vi "CODCr数据插入DATA (子VI).vi"(11 "Enum输入":refnum<vi>) -> (3 "data":T1)   [LabVIEW 2016, in "CODCr库.lvlib"]
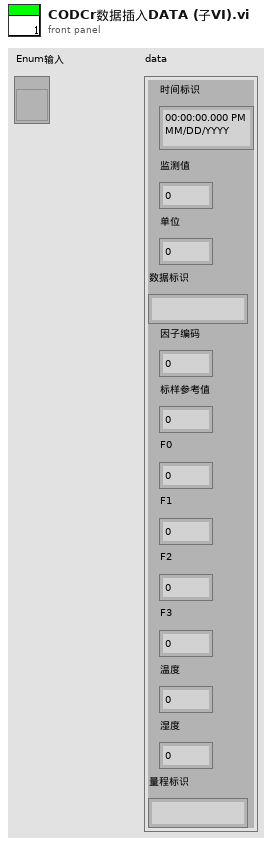
[diagram p1: front panel]
types:
  T1 = cluster{"时间标识":timestamp, "监测值":sgl, "单位":u16, "数据标识":string, "因子编码":u32, "标样参考值":sgl, "F0":sgl, "F1":sgl, "F2":sgl, "F3":sgl, "温度":sgl, "湿度":sgl, "量程标识":string}
  T2 = cluster{"系统时间":timestamp, "工作状态":u16, "测量模式":u16, "告警代码":enum16{"无告警", "缺试剂告警", "缺水样告警", "缺蒸馏水告警", "缺标液告警", "仪表漏液告警", "标定异常告警", "超量程告警", "加热异常", "低试剂预警", "超上限告警", "超下限告警", "仪表内部其他异常", "滴定异常告警", "电极异常告警", "量程切换告警", "参数设置告警", "PH电极电位异常", "电导率电极异常", "浊度光度异常", "溶解氧电极异常", "溶解氧光强异常", "温度异常告警", "PH异常告警", "溶解氧异常告警", "电导率异常告警", "浊度异常告警", "叶绿素异常告警", "藻密度异常告警", "蓝绿藻异常告警", "ORP异常告警", "氨氮异常告警", "清洁刷异常告警", "SD卡异常告警", "蓝牙异常告警", "Wifi异常告警", "流程异常告警"}, "故障代码":enum16{"无故障", "电机故障", "温度故障", "通讯故障", "滴定故障"}, "日志代码":u16, "软件版本":u16, "F0":sgl, "F1":sgl, "F2":sgl, "F3":sgl, "T":sgl, "H":sgl, "id":u16, "flowid":u16, "量程":u16}
  T3 = cluster{"因子编码":u32, "单位":u16, "标样参考值":sgl, "水样数据时间":timestamp, "水样实测值":sgl, "水样数据标识":string, "标样数据时间":timestamp, "标样实测值":sgl, "标样数据标识":string, "空白数据时间":timestamp, "空白实测值":sgl, "空白数据标识":string, "零点核查数据时间":timestamp, "零点核查实测值":sgl, "零点核查数据标识":string, "跨度核查数据时间":timestamp, "跨度核查实测值":sgl, "跨度核查数据标识":string, "加标回收数据时间":timestamp, "加标回收实测值":sgl, "加标回收数据标识":string, "平行样数据时间":timestamp, "平行样实测值":sgl, "平行样数据标识":string}
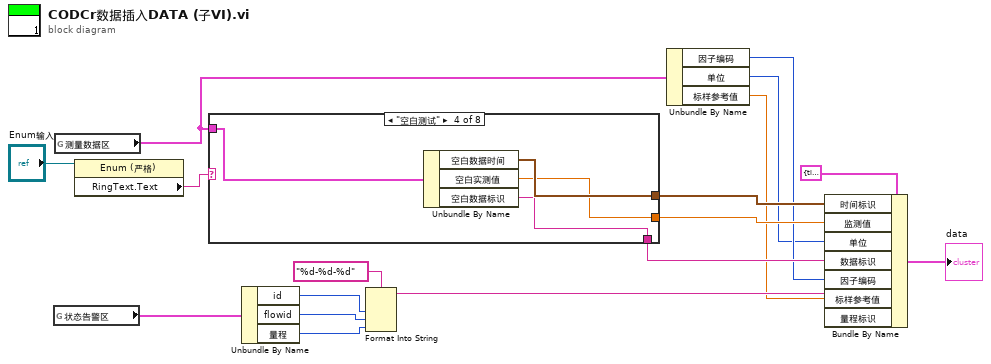
[diagram p0: block diagram]
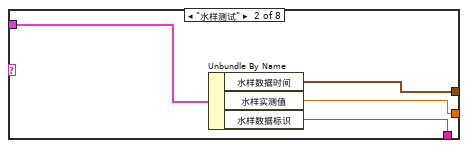
[diagram p3: hidden frame]
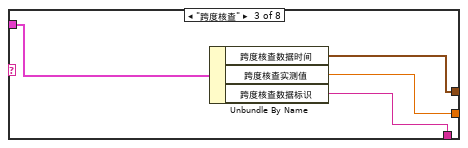
[diagram p4: hidden frame]
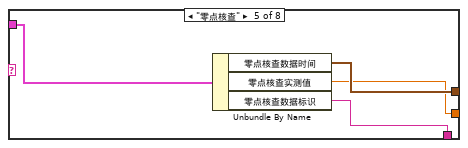
[diagram p5: hidden frame]
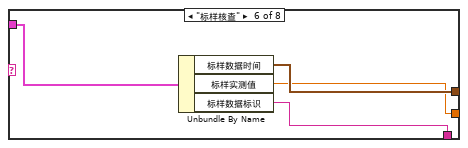
[diagram p6: hidden frame]
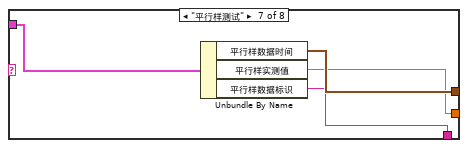
[diagram p7: hidden frame]
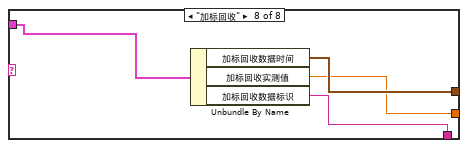
[diagram p8: hidden frame]
diagram:
  n1 = global read "CODcr全局变量.vi" "状态告警区"() -> (w2:T2)
  n2 = global read "CODcr全局变量.vi" "测量数据区"() -> (w1:T3)
  n3 = property on="属性节点" class="Enum (严格)"(reference="Enum输入") -> ("RingText.Text"=w6:string)  [unwired: 1 in, 2 out]
  n4 = case shown="\"空白测试\"" w6 {
    tunnel: w1 -> [_ w21 w25 w29 w33 w34 w38 w42]
    tunnel: [_ w20 w24 w28 w32 w37 w41 w45] -> w15
    tunnel: [_ w19 w23 w27 w31 w36 w40 w44] -> w16
    tunnel: [_ w18 w22 w26 w30 w35 w39 w43] -> w17
    frame "假", Default {
    }
    frame "水样测试" {
      n5 = Unbundle By Name(w21) -> ("水样数据时间"=w20:timestamp, "水样实测值"=w19:sgl, "水样数据标识"=w18:string)
    }
    frame "跨度核查" {
      n6 = Unbundle By Name(w25) -> ("跨度核查数据时间"=w24:timestamp, "跨度核查实测值"=w23:sgl, "跨度核查数据标识"=w22:string)
    }
    frame "空白测试" {
      n7 = Unbundle By Name(w29) -> ("空白数据时间"=w28:timestamp, "空白实测值"=w27:sgl, "空白数据标识"=w26:string)
    }
    frame "零点核查" {
      n8 = Unbundle By Name(w33) -> ("零点核查数据时间"=w32:timestamp, "零点核查实测值"=w31:sgl, "零点核查数据标识"=w30:string)
    }
    frame "标样核查" {
      n9 = Unbundle By Name(w34) -> ("标样数据时间"=w37:timestamp, "标样实测值"=w36:sgl, "标样数据标识"=w35:string)
    }
    frame "平行样测试" {
      n10 = Unbundle By Name(w38) -> ("平行样数据时间"=w41:timestamp, "平行样实测值"=w40:sgl, "平行样数据标识"=w39:string)
    }
    frame "加标回收" {
      n11 = Unbundle By Name(w42) -> ("加标回收数据时间"=w45:timestamp, "加标回收实测值"=w44:sgl, "加标回收数据标识"=w43:string)
    }
  }
  n12 = Unbundle By Name(w2) -> ("id"=w11:u16, "flowid"=w12:u16, "量程"=w13:u16)
  n13 = Format Into String(format string="%d-%d-%d" ("格式字符串"), w11, w12, w13) -> (resulting string=w14:string)  [unwired: 2 in, 1 out]
  n14 = Unbundle By Name(w1) -> ("因子编码"=w8:u32, "单位"=w7:u16, "标样参考值"=w9:sgl)
  n15 = Bundle By Name(cluster=T1 {"时间标识"=timestamp(0 s since 1904-01-01), "监测值"=0.0, "单位"=0, "数据标识"="", "因子编码"=0, "标样参考值"=0.0, "F0"=0.0, "F1"=0.0, "F2"=0.0, "F3"=0.0, "温度"=0.0, "湿度"=0.0, "量程标识"=""} ("data"), "时间标识"=w15, "监测值"=w16, "单位"=w7, "数据标识"=w17, "因子编码"=w8, "标样参考值"=w9, "量程标识"=w14) -> (→"data":T1)
